vi "Start Log.vi"(8 "error in (no error)":errorcluster, 10 "Data":T1, 11 "Log Manager Module in":refnum<class "Log Manager Module.lvclass">) -> (0 "error out":errorcluster, 3 "Log Manager Module out":refnum<class "Log Manager Module.lvclass">)   [LabVIEW 2020, in "VolatusData.lvlib" / "Log Manager Module.lvclass"]
uses:
  Log Manager Module.lvclass
  C:/dev/lv20CE/relink/lv-volatus/Volatus/Module/Module.lvclass
  messages/StartLog/Data.ctl
  Log Manager Module.lvclass/Log Manager Module.ctl
  Volatus/Module/Module.lvclass/Module.ctl
  Logging State.ctl
  Volatus/Module/Module.lvclass
  VolatusData.lvlib
  messages/StartLog/StartLog.lvlib
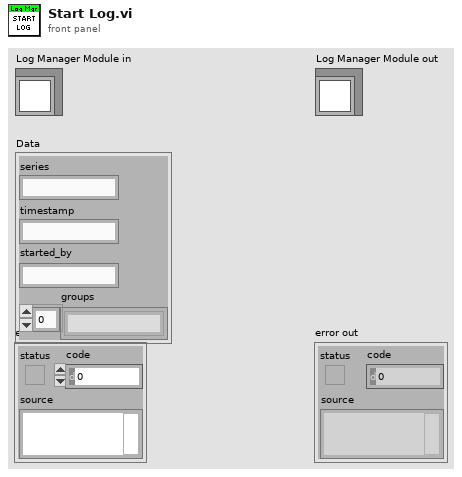
[diagram p1: front panel]
types:
  T1 = typedef "StartLog.lvlib/Data.ctl" = cluster{"series":string, "timestamp":string, "started_by":string, "groups":string[]}
  T2 = typedef "VolatusData.lvlib/Logging State.ctl" = enum16{"Idle", "Starting", "Logging", "Stopping"}
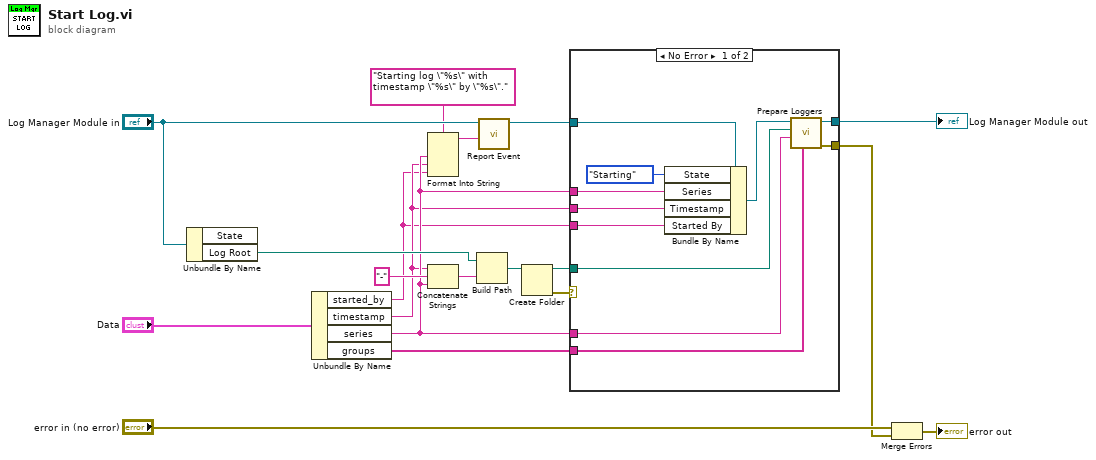
[diagram p0: block diagram]
diagram:
  n1 = Unbundle By Name("Log Manager Module in") -> ("Log Root"=w16:path)  [unwired: 1 out]
  n2 = Unbundle By Name("Data") -> ("started_by"=w2:string, "timestamp"=w3:string, "series"=w4:string, "groups"=w1:string[])
  n3 = Format Into String(format string="Starting log \"%s\" with timestamp \"%s\" by \"%s\".", w4, w3, w2) -> (resulting string=w5:string)  [unwired: 2 in, 1 out]
  n4 = Concatenate Strings(w3, "-" ("string"), w4) -> (w11:string)
  n5 = Build Path(base path=w16, name or relative path=w11) -> (appended path=w10:path)
  n6 = call "Report Event.vi"("Message"=w5, "Module in"="Log Manager Module in") -> ("Module out"=w7:refnum<class "Log Manager Module.lvclass">)  [unwired: 8 in, 1 out]
  n7 = Create Folder(path (use dialog)=w10) -> (created path=w8:path, error out=w9:errorcluster)  [unwired: 2 in, 1 out]
  n8 = case shown="No Error" w9 {
    selector: w9 -> [_ w32]
    tunnel: w7 -> [w29 w31]
    tunnel: w8 -> [w24 _]
    tunnel: w4 -> [w25 _]
    tunnel: [w28 w31] -> w15
    tunnel: [w26 w32] -> w13
    tunnel: w4 -> [w23 _]
    tunnel: w3 -> [w22 _]
    tunnel: w2 -> [w21 _]
    tunnel: w1 -> [w20 _]
    frame No Error {
      n9 = Bundle By Name(cluster=w29, "State"=Logging_State."Starting" ("Logging State"), "Series"=w23, "Timestamp"=w22, "Started By"=w21) -> (w27:refnum<class "Log Manager Module.lvclass">)
      n10 = call "Prepare Loggers.vi"("Groups"=w20, "Series"=w25, "Folder"=w24, "Log Manager Module in"=w27) -> ("error out"=w26:errorcluster, "Log Manager Module out"=w28:refnum<class "Log Manager Module.lvclass">)  [unwired: 6 in]
    }
    frame Error {
    }
  }
  "Log Manager Module out" <- w15
  n11 = Merge Errors("error in (no error)", w13) -> (→"error out":errorcluster)
